vi "String to Path.vi"(1 "String":string) -> (0 "Path":path)   [LabVIEW 2017, in "CSM Shared.lvlib"]
uses:
  CSM Shared.lvlib
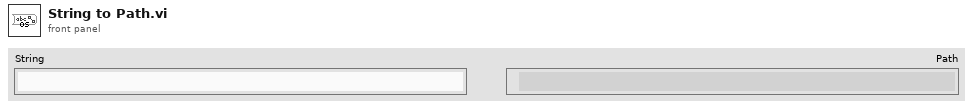
[diagram p1: front panel]
types:
  T1 = enum16{"Absolute path", "Relative path", "Not-a-path"}
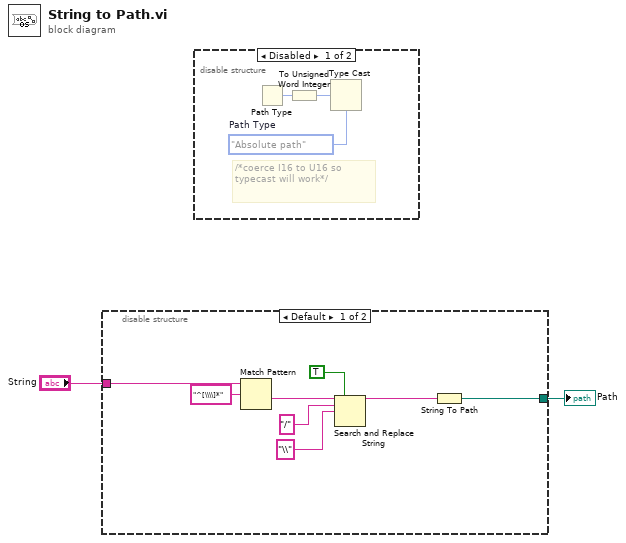
[diagram p0: block diagram]
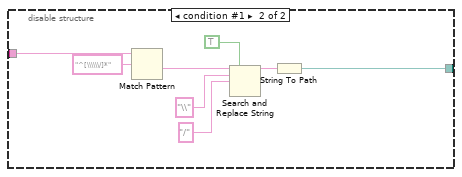
[diagram p3: hidden frame]
diagram:
  n1 = disable-structure shown="Default" {
    disable-tunnel: [w10 w11] -> w2
    disable-tunnel: "String" -> [w9 w17]
    frame condition #0 (active) {
      n2 = Match Pattern(string=w9, regular expression="^[\\\\]*") -> (after substring=w6:string)  [unwired: 1 in, 3 out]
      n3 = Search and Replace String(replace all?=TRUE ("replace all? (F)"), input string=w6, search string="/" ("regular expression"), replace string="\\" ("regular expression")) -> (result string=w5:string)  [unwired: 4 in, 3 out]
      n4 = String To Path(string=w5) -> (path=w10:path)
    }
    frame condition #1 {
      n5 = Match Pattern(string=w17, regular expression="^[\\\\\\/]*") -> (after substring=w16:string)  [unwired: 1 in, 3 out]
      n6 = Search and Replace String(replace all?=TRUE ("replace all? (F)"), input string=w16, search string="\\" ("regular expression"), replace string="/" ("regular expression")) -> (result string=w12:string)  [unwired: 4 in, 3 out]
      n7 = String To Path(string=w12) -> (path=w11:path)
    }
  }
  "Path" <- w2
  n8 = disable-structure shown="Disabled" {
    frame Disabled {
      w20 = T1."Absolute path"  # Path Type
      # "/*coerce I16 to U16 so typecast will work*/"
      n9 = Path Type() -> (0:w19:i16)  [unwired: 1 in]
      n10 = To Unsigned Word Integer(number=w19) -> (unsigned 16bit integer=w21:u16)
      n11 = Type Cast(type=w20, x=w21) -> ()  [unwired: 1 out]
    }
    frame Enabled {
    }
  }
